vi "myRIO-1900 Customized FPGA.vi"() -> ()   [LabVIEW 2013]
doc: "This VI contains the NI myRIO FPGA shipping personality. This VI compiles and runs on the NI myRIO FPGA target. You can modify this VI to suit your application needs. National Instruments recommends that you only add new FPGA code to this VI and do not modify the existing code. This VI might not work correctly with the myRIO VIs if you modify the existing code."
uses:
  Sub VIs/Utilities/Start Boolean.ctl
  <vilib>/Platform/TimedLoop/XDataNode/timing_clust.ctl
  <vilib>/Platform/TimedLoop/XDataNode/nitl_modes.ctl
  <vilib>/Platform/TimedLoop/XDataNode/wakeup.ctl
  <vilib>/rvi/Emulation/niFpgaSctlEmulationGetInTimedLoop.vi
  <vilib>/rvi/Emulation/niFpgaEmulationReportErrorSimple.vi
  <vilib>/rvi/Emulation/niFpgaGetClockAttributes.vi
  <vilib>/rvi/Emulation/niFpgaCriticalErrorInLSC.vi
  <vilib>/rvi/eio/common/nirviEmuTemplateMethod_errors.vi
  <vilib>/rvi/eio/common/nirviEmuTemplatePropertyGet_noerrors.vi
  <vilib>/Platform/TimedLoop/XDataNode/XDataNode.xnode
  <vilib>/eio/EIONode/EIONode.xnode
  <vilib>/eio/EIOPropertyNode/EIOPropertyNode.xnode
  <vilib>/Platform/TimedLoop/XDataNode/XDNodeRunTimeDep.lvlib
  <vilib>/rvi/eio/common/nirviEmuTemplatePropertyGet_errors.vi
  <vilib>/rvi/eio/common/nirviEmuTemplatePropertySet_errors.vi
  <vilib>/rvi/eio/common/nirviEmuTemplatePropertySet_noerrors.vi
panel:
  out "Sonar Error 2":bool
  out "Sonar Timed Out 2":bool
  out "Sonar Reading 2":i32
  out "Sonar Error 1":bool
  out "Sonar Timed Out 1":bool
  out "Sonar Reading 1":i32
  out "Sonar Error 0":bool
  out "Sonar Timed Out 0":bool
  out "Sonar Reading 0":i32
  out "ACC.SCALE.WGHT":u16
  out "SYS.ACC_SCALE.RDY":bool
  out "AO.SYS.STAT":bool
  out "AI.B_1.WGHT":u32
  out "AO.B_0.WGHT":u32
  out "AO.B_1.WGHT":u32
  out "AO.B_0.OFST":u32
  out "AO.B_1.OFST":u32
  out "AO.A_0.WGHT":u32
  out "AO.A_1.WGHT":u32
  out "AO.C_0.WGHT":u32
  out "AO.C_1.WGHT":u32
  out "AO.AudioOut_L.WGHT":u32
  out "AO.AudioOut_R.WGHT":u32
  out "AO.A_0.OFST":u32
  out "AO.C_0.OFST":u32
  out "AO.C_1.OFST":u32
  out "AO.AudioOut_L.OFST":u32
  out "AO.AudioOut_R.OFST":u32
  out "AO.A_1.OFST":u32
  out "SYS.AO_SCALE.RDY":bool
  out "SYS.AI_SCALE.RDY":bool
  out "AI.A_1.OFST":u32
  out "AI.A_2.OFST":u32
  out "AI.A_3.OFST":u32
  out "AI.B_0.OFST":u32
  out "AI.B_1.OFST":u32
  out "AI.B_2.OFST":u32
  out "AI.B_3.OFST":u32
  out "AI.C_0.OFST":u32
  out "AI.C_1.OFST":u32
  out "AI.AudioIn_L.OFST":u32
  out "AI.AudioIn_R.OFST":u32
  out "AI.A_0.OFST":u32
  out "AI.AudioIn_R.WGHT":u32
  out "AI.AudioIn_L.WGHT":u32
  out "AI.C_1.WGHT":u32
  out "AI.C_0.WGHT":u32
  out "AI.B_3.WGHT":u32
  out "AI.B_2.WGHT":u32
  out "AI.B_0.WGHT":u32
  out "AI.A_3.WGHT":u32
  out "AI.A_2.WGHT":u32
  out "AI.A_1.WGHT":u32
  out "AI.A_0.WGHT":u32
  in  "DO.LED3:0":u8 format="%04b"
  out "ACC.Z.VAL":u16
  out "SYS.ACC.RDY":bool
  out "ACC.Y.VAL":u16
  out "ACC.X.VAL":u16
  in  "AO.SYS.GO":T1
  in  "AO.AudioOut_L.VAL":u16
  in  "AO.AudioOut_R.VAL":u16
  out "AI.AudioIn_L.VAL":u16
  out "AI.AudioIn_R.VAL":u16
  in  "DIO.B_15:8.OUT":u8 format="%08b"
  in  "DIO.B_15:8.DIR":u8 format="%08b"
  out "DIO.B_15:8.IN":u8 format="%08b"
  in  "DIO.A_15:8.DIR":u8 format="%08b"
  in  "DIO.A_15:8.OUT":u8 format="%08b"
  out "DIO.A_15:8.IN":u8 format="%08b"
  in  "PWM.C_0.MAX":u16
  in  "PWM.C_0.CMP":u16
  out "PWM.C_0.CNTR":u16
  in  "PWM.C_0.CNFG":u8 format="%08b"
  in  "PWM.C_0.CS":u8
  in  "PWM.C_1.MAX":u16
  in  "PWM.C_1.CMP":u16
  out "PWM.C_1.CNTR":u16
  in  "PWM.C_1.CNFG":u8 format="%08b"
  in  "PWM.C_1.CS":u8
  out "ENC.C_1.STAT":u8 format="%08b"
  out "ENC.C_1.CNTR":u32
  in  "ENC.C_1.CNFG":u8 format="%08b"
  out "ENC.C_0.STAT":u8 format="%08b"
  out "ENC.C_0.CNTR":u32
  in  "ENC.C_0.CNFG":u8 format="%08b"
  in  "SYS.SELECTA":u8 format="%08b"
  in  "SYS.SELECTC":u8 format="%08b"
  in  "SYS.SELECTB":u8 format="%08b"
  in  "AO.C_1.VAL":u16
  in  "AO.C_0.VAL":u16
  out "AI.C_0.VAL":u16
  out "AI.C_1.VAL":u16
  in  "DIO.C_7:0.OUT":u8 format="%08b"
  in  "DIO.C_7:0.DIR":u8 format="%08b"
  out "DIO.C_7:0.IN":u8 format="%08b"
  in  "DIO.A_7:0.DIR":u8 format="%08b"
  in  "DIO.A_7:0.OUT":u8 format="%08b"
  out "DIO.A_7:0.IN":u8 format="%08b"
  in  "PWM.B_0.CMP":u16
  in  "PWM.B_0.MAX":u16
  out "PWM.B_0.CNTR":u16
  in  "PWM.B_0.CNFG":u8 format="%08b"
  in  "PWM.B_0.CS":u8
  in  "PWM.B_1.CMP":u16
  in  "PWM.B_1.MAX":u16
  out "PWM.B_1.CNTR":u16
  in  "PWM.B_1.CNFG":u8 format="%08b"
  in  "PWM.B_1.CS":u8
  in  "PWM.B_2.CMP":u16
  in  "PWM.B_2.MAX":u16
  out "PWM.B_2.CNTR":u16
  in  "PWM.B_2.CNFG":u8 format="%08b"
  in  "PWM.B_2.CS":u8
  out "SYS.RDY":bool
  out "SYS.AI.RDY":bool
  in  "I2C.B.GO":T1
  in  "I2C.B.CNFG":u8 format="%08b"
  in  "I2C.B.DATO":u8
  out "I2C.B.DATI":u8
  in  "I2C.B.ADDR":u8 format="%08.0f"
  in  "I2C.B.CNTR":u8
  in  "I2C.B.CNTL":u8 format="%08b"
  out "I2C.B.STAT":u8 format="%08b"
  out "SPI.B.STAT":u8 format="%08b"
  in  "SPI.B.GO":T1
  out "SPI.A.STAT":u8 format="%08b"
  in  "SPI.A.GO":T1
  out "ENC.B.STAT":u8 format="%08b"
  out "ENC.A.STAT":u8 format="%08b"
  out "ENC.B.CNTR":u32
  out "ENC.A.CNTR":u32
  in  "ENC.B.CNFG":u8 format="%08b"
  in  "ENC.A.CNFG":u8 format="%08b"
  in  "SPI.B.DATO":u16
  out "SPI.B.DATI":u16
  in  "SPI.B.CNFG":u16 format="%016.0f"
  in  "SPI.B.CNT":u16
  in  "SPI.A.CNT":u16
  in  "SPI.A.CNFG":u16 format="%016b"
  out "SPI.A.DATI":u16
  in  "SPI.A.DATO":u16
  in  "PWM.A_0.MAX":u16
  in  "PWM.A_0.CMP":u16
  out "PWM.A_0.CNTR":u16
  in  "PWM.A_0.CNFG":u8 format="%08b"
  in  "PWM.A_0.CS":u8
  in  "PWM.A_1.CMP":u16
  in  "PWM.A_1.MAX":u16
  out "PWM.A_1.CNTR":u16
  in  "PWM.A_1.CNFG":u8 format="%08b"
  in  "PWM.A_1.CS":u8
  in  "PWM.A_2.CMP":u16
  in  "PWM.A_2.MAX":u16
  out "PWM.A_2.CNTR":u16
  in  "PWM.A_2.CNFG":u8 format="%08b"
  in  "PWM.A_2.CS":u8
  in  "DIO.B_7:0.OUT":u8 format="%08b"
  in  "DIO.B_7:0.DIR":u8 format="%08b"
  out "DIO.B_7:0.IN":u8 format="%08b"
  out "AI.A_0.VAL":u16
  out "AI.A_1.VAL":u16
  out "AI.A_2.VAL":u16
  out "AI.A_3.VAL":u16
  out "AI.B_0.VAL":u16
  out "AI.B_1.VAL":u16
  out "AI.B_2.VAL":u16
  out "AI.B_3.VAL":u16
  in  "AO.B_1.VAL":u16
  in  "AO.B_0.VAL":u16
  in  "AO.A_1.VAL":u16
  in  "AO.A_0.VAL":u16
  # "System"
  # "Onboard Devices"
  # "Connector A"
  # "Connector B"
  # "Connector C"
  # "Audio Connector"
  # "Accelerometer"
  # "Analog Input"
  # "Analog Output"
  # "Digital I/O"
  # "Counters / PWM"
  # "SPI Master"
  # "Analog Input"
  # "Analog Output"
  # "Digital I/O"
  # "Counters / PWM"
  # "SPI Master"
  # "Analog Input"
  # "Analog Output"
  # "Digital I/O"
  # "Counters / PWM"
  # "Analog Input"
  # "Encoders"
  # "Buttons & LEDs"
  # "I2C Master"
  # "I2C Master"
  # "Encoders"
  # "Encoders"
  # "Analog Output"
  # "IO Configuration"
  # "IO Configuration"
  # "IO Configuration"
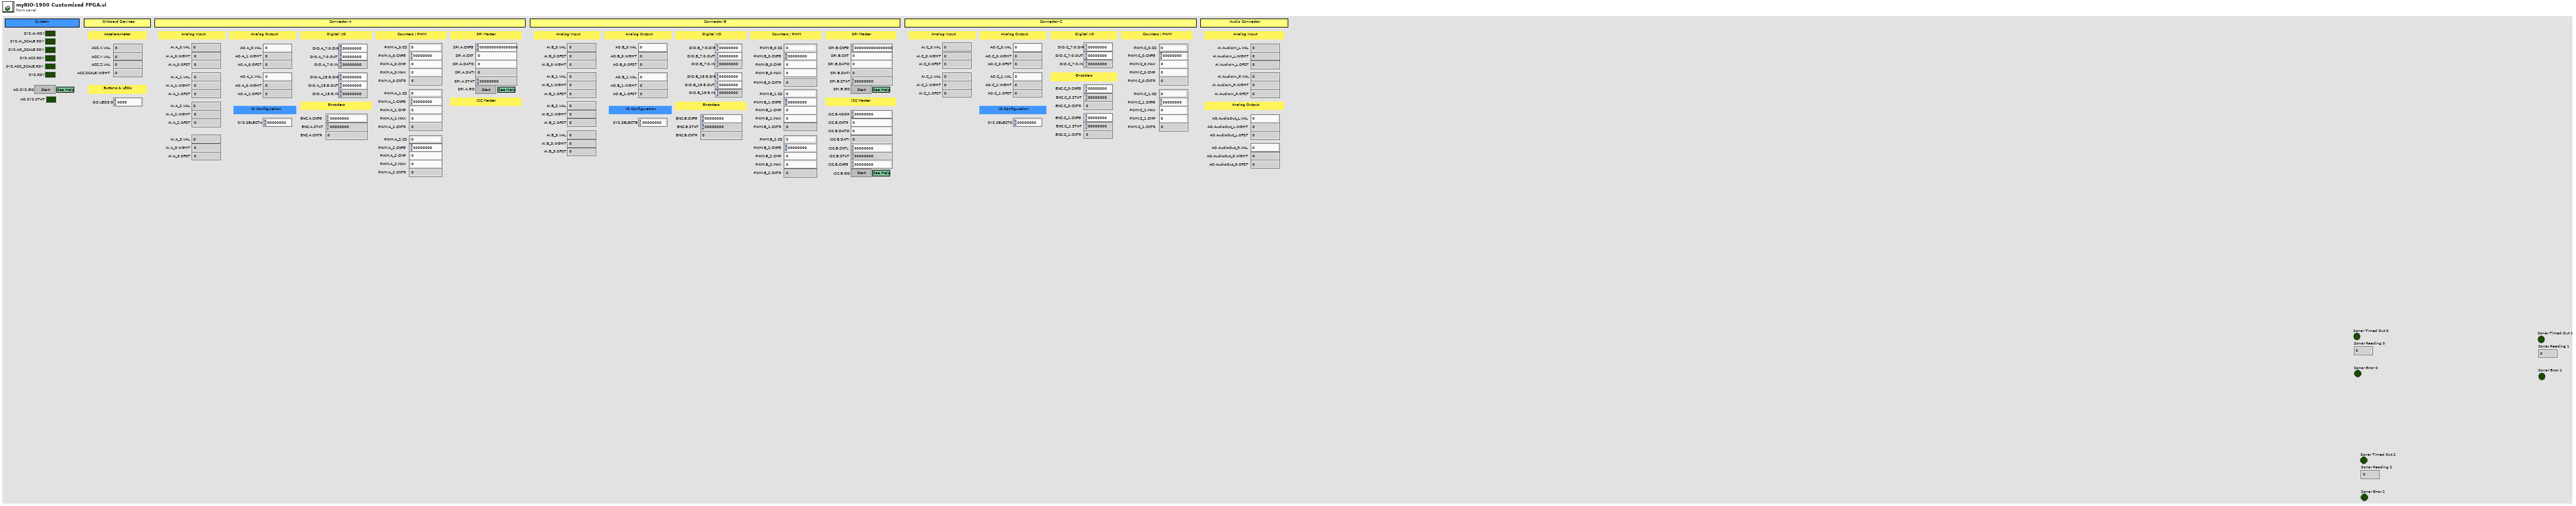
[diagram p1: front panel]
types:
  T1 = typedef "Start Boolean.ctl" = bool
  T2 = typedef "XDNodeRunTimeDep.lvlib/timing_clust.ctl" = cluster{"Expected End [f-1]":u64, "Actual End [f-1]":u64, "Finished Late? [f-1]":bool, "Expected End [i-1]":u64, "Actual End [i-1]":u64, "Finished Late? [i-1]":bool, "Expected Start [i]":u64, "Actual Start [i]":u64, "Expected Start [f]":u64, "Actual Start [f]":u64, "Source Name":string, "Structure Name":string, "Period":i64, "Deadline":i64, "Offset":i64, "Start":i64, "Priority":i32, "Timeout":i32, "Mode":T3, "Wakeup Reason":T4, "Error":errorcluster, "Source Type":string, "Secondary Source Type":string, "Global End Time":u64, "Global Start Time":u64, "Frame Duration":u64, "Iteration Duration":u64, "Assigned CPU":i32, "I/O Scan Engine Mode":u32}
  T3 = typedef "XDNodeRunTimeDep.lvlib/nitl_modes.ctl" = enum32{"No Change", "Process missed periods, maintain original phase", "Discard missed periods, maintain original phase", "Process missed periods, ignore original phase", "Discard missed periods, ignore original phase"}
  T4 = typedef "XDNodeRunTimeDep.lvlib/wakeup.ctl" = enum32{"Normal", "Aborted", "Asynchronous wakeup", "Timing source error", "Timed loop error", "Timeout"}
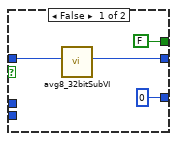
[diagram p2: hidden frame]
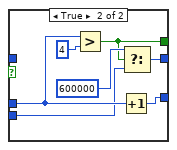
[diagram p3: hidden frame]
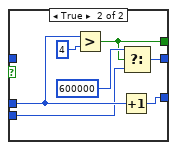
[diagram p4: hidden frame]
diagram:
  # "NOTE: The SYS.RDY boolean MUST exist and must become TRUE at some point otherwise the myRIO API will not function correctly."
  # "All DIO operations occur inside one single cycle timed loop (SCTL) since the IO is shared."
  # "The analog input scaling values are stored on the hardware. The RDY boolean should be checked before the values are used otherwise the analog input vlaues could be scaled incorrectly.\n\nAfter the first iteration of the while loop, all indicators have valid values."
  # "The analog output scaling values are stored on the hardware. The RDY boolean should be checked before the values are used otherwise the analog output vlaues could be scaled incorrectly.\n\nAfter the first iteration of the while loop, all indicators have valid values."
  # "The accelerometer nodes takes some time before the values can first be read (this is due to the time taken to read from the acceleromter). An iteration of the while loop will not complete until the accelerometer values have been read.\n\nAfter the first iteration of the while loop, all indicators have valid values."
  # "The onboard accelerometer has a range of +/- 8g which translates to 256 bits/g. The scaling weight is hardcoded in the FPGA to allow for future updates with minimal changes in the myRIO code. The RDY boolean should be checked before the values are used otherwise the analog output vlaues could be scaled incorrectly.\n\nAfter the first iteration of the while loop, all indicators have valid values."
  # "Onboard Accelerometer Scaling"
  # "Analog Output Scaling Constants"
  # "Analog Input Scaling Constants"
  # "Onboard Accelerometer"
  # "Onboard DIO"
  # "Connector B DIO"
  # "There is some delay between when the FPGA code starts and the analog inputs, accelerometer, and scaling values outputs are valid. If the host wants to ensure that there are valid values in theses registers it should wait for each subsystem to finish its initialization process. \n\nWhen all subsystems have finished initializinig, the SYS.RDY indicator will be true, which can be polled by the host to determine the status of the FPGA. Alternatively, the host can poll the individual SYS.xx.RDY indicators to determine the status of the individual subsystems.\n\nThis loop continues indefinitely, essentially making SYS.RDY a read-only register."
  # "The analog input nodes takes some time before the values can first be read (this is due to the time taken to setup the ADC and convert the first reading). An iteration of the while loop will not complete until all the analog input channels have been sampled.\n\nAfter the first iteration of the while loop, all indicators have valid values."
  # "Note: On some hardware a \"ghosting effect\" may occur on any unconnected AI channels. For example, if channel AI0 is connected and channels AI1 - AI7 are not connected the the value read at AI0 may be seen on indicators AI1 - AI7. This is common for hardware that use a multiplexed (MUXed) Analog-to-Digital converter (ADC) since the input analog signal is used to charge a capacitor which does not discharge before the unconnected channel is read.\n\n\"Ghosting\" effect can be hidden be using an mask register which will be used to decide when the indicator should be updated."
  # "The analog output nodes take some time before values are written to the pins. The GO and STAT registers are used to handshake between the FPGA and host. When the host wants the values to be written it sets the GO register to true. If the host reads the STAT register before setting GO, it can then wait for the STAT register value to invert which will tell the host that the output values have been written."
  # "Connector A DIO"
  # "Connector C  DIO"
  # "Host Synchronization"
  # "Analog Output"
  # "Analog Input"
  n1 = while {
    stop <- FALSE stop-if-true
    n2 = local read "SYS.ACC_SCALE.RDY"() -> (w10:bool)
    n3 = local read "SYS.AO_SCALE.RDY"() -> (w11:bool)
    n4 = local read "SYS.AI_SCALE.RDY"() -> (w12:bool)
    n5 = local read "SYS.ACC.RDY"() -> (w13:bool)
    n6 = local read "SYS.AI.RDY"() -> (w15:bool)
    n7 = Compound Arithmetic op=AND(w15, w13, w12, w11, w10) -> (→"SYS.RDY":bool)
  }
  n8 = while {
    i -> [w27]
    stop <- FALSE stop-if-true
    n9 = xnode "FPGA I/O Node"() -> ("ConnectorA/AI0"=→"AI.A_0.VAL":u16, "ConnectorA/AI1"=→"AI.A_1.VAL":u16, "ConnectorA/AI2"=→"AI.A_2.VAL":u16, "ConnectorA/AI3"=→"AI.A_3.VAL":u16, "ConnectorB/AI0"=→"AI.B_0.VAL":u16, "ConnectorB/AI1"=→"AI.B_1.VAL":u16, "ConnectorB/AI2"=→"AI.B_2.VAL":u16, "ConnectorB/AI3"=→"AI.B_3.VAL":u16, "ConnectorC/AI0"=w21:i16, "ConnectorC/AI1"=w20:i16, "AudioIn/Left"=w19:i16, "AudioIn/Right"=w18:i16)  [unwired: 12 in, 12 out]
    n10 = Greater Than 0?(x=w27) -> (x > 0?=→"SYS.AI.RDY":bool)
    n11 = To Unsigned Word Integer(number=w21) -> (unsigned 16bit integer=→"AI.C_0.VAL":u16)
    n12 = To Unsigned Word Integer(number=w20) -> (unsigned 16bit integer=→"AI.C_1.VAL":u16)
    n13 = To Unsigned Word Integer(number=w19) -> (unsigned 16bit integer=→"AI.AudioIn_L.VAL":u16)
    n14 = To Unsigned Word Integer(number=w18) -> (unsigned 16bit integer=→"AI.AudioIn_R.VAL":u16)
  }
  n15 = while {
    i -> [w37]
    stop <- FALSE stop-if-true
    n16 = Greater Than 0?(x=w37) -> (x > 0?=→"SYS.AI_SCALE.RDY":bool)
    n17 = xnode "FPGA I/O Property Node"("FPGA I/O In"=refnum<k21> "ConnectorA/AI0" ("FPGA I/O")) -> ("LSB Weight"=→"AI.A_0.WGHT":u32, "Offset"=w62:i32)  [unwired: 1 out]
    n18 = xnode "FPGA I/O Property Node"("FPGA I/O In"=refnum<k21> "ConnectorA/AI1" ("FPGA I/O")) -> ("LSB Weight"=→"AI.A_1.WGHT":u32, "Offset"=w50:i32)  [unwired: 1 out]
    n19 = xnode "FPGA I/O Property Node"("FPGA I/O In"=refnum<k21> "ConnectorA/AI2" ("FPGA I/O")) -> ("LSB Weight"=→"AI.A_2.WGHT":u32, "Offset"=w59:i32)  [unwired: 1 out]
    n20 = xnode "FPGA I/O Property Node"("FPGA I/O In"=refnum<k21> "ConnectorA/AI3" ("FPGA I/O")) -> ("LSB Weight"=→"AI.A_3.WGHT":u32, "Offset"=w58:i32)  [unwired: 1 out]
    n21 = xnode "FPGA I/O Property Node"("FPGA I/O In"=refnum<k21> "ConnectorB/AI0" ("FPGA I/O")) -> ("LSB Weight"=→"AI.B_0.WGHT":u32, "Offset"=w57:i32)  [unwired: 1 out]
    n22 = xnode "FPGA I/O Property Node"("FPGA I/O In"=refnum<k21> "ConnectorB/AI1" ("FPGA I/O")) -> ("LSB Weight"=→"AI.B_1.WGHT":u32, "Offset"=w56:i32)  [unwired: 1 out]
    n23 = xnode "FPGA I/O Property Node"("FPGA I/O In"=refnum<k21> "ConnectorB/AI2" ("FPGA I/O")) -> ("LSB Weight"=→"AI.B_2.WGHT":u32, "Offset"=w55:i32)  [unwired: 1 out]
    n24 = xnode "FPGA I/O Property Node"("FPGA I/O In"=refnum<k21> "ConnectorB/AI3" ("FPGA I/O")) -> ("LSB Weight"=→"AI.B_3.WGHT":u32, "Offset"=w54:i32)  [unwired: 1 out]
    n25 = xnode "FPGA I/O Property Node"("FPGA I/O In"=refnum<k21> "ConnectorC/AI0" ("FPGA I/O")) -> ("LSB Weight"=→"AI.C_0.WGHT":u32, "Offset"=w53:i32)  [unwired: 1 out]
    n26 = xnode "FPGA I/O Property Node"("FPGA I/O In"=refnum<k21> "ConnectorC/AI1" ("FPGA I/O")) -> ("LSB Weight"=→"AI.C_1.WGHT":u32, "Offset"=w52:i32)  [unwired: 1 out]
    n27 = xnode "FPGA I/O Property Node"("FPGA I/O In"=refnum<k21> "AudioIn/Left" ("FPGA I/O")) -> ("LSB Weight"=→"AI.AudioIn_L.WGHT":u32, "Offset"=w51:i32)  [unwired: 1 out]
    n28 = xnode "FPGA I/O Property Node"("FPGA I/O In"=refnum<k21> "AudioIn/Right" ("FPGA I/O")) -> ("LSB Weight"=→"AI.AudioIn_R.WGHT":u32, "Offset"=w61:i32)  [unwired: 1 out]
    n29 = To Unsigned Long Integer(number=w62) -> (unsigned 32bit integer=→"AI.A_0.OFST":u32)
    n30 = To Unsigned Long Integer(number=w50) -> (unsigned 32bit integer=→"AI.A_1.OFST":u32)
    n31 = To Unsigned Long Integer(number=w59) -> (unsigned 32bit integer=→"AI.A_2.OFST":u32)
    n32 = To Unsigned Long Integer(number=w58) -> (unsigned 32bit integer=→"AI.A_3.OFST":u32)
    n33 = To Unsigned Long Integer(number=w57) -> (unsigned 32bit integer=→"AI.B_0.OFST":u32)
    n34 = To Unsigned Long Integer(number=w56) -> (unsigned 32bit integer=→"AI.B_1.OFST":u32)
    n35 = To Unsigned Long Integer(number=w55) -> (unsigned 32bit integer=→"AI.B_2.OFST":u32)
    n36 = To Unsigned Long Integer(number=w54) -> (unsigned 32bit integer=→"AI.B_3.OFST":u32)
    n37 = To Unsigned Long Integer(number=w53) -> (unsigned 32bit integer=→"AI.C_0.OFST":u32)
    n38 = To Unsigned Long Integer(number=w52) -> (unsigned 32bit integer=→"AI.C_1.OFST":u32)
    n39 = To Unsigned Long Integer(number=w51) -> (unsigned 32bit integer=→"AI.AudioIn_L.OFST":u32)
    n40 = To Unsigned Long Integer(number=w61) -> (unsigned 32bit integer=→"AI.AudioIn_R.OFST":u32)
  }
  n41 = while {
    stop <- FALSE stop-if-true
    n42 = feedback #1(FALSE) -> (w88:bool)
    n43 = case shown="True" "AO.SYS.GO" {
      tunnel: "AO.C_0.VAL" -> [_ w110]
      tunnel: "AO.C_1.VAL" -> [_ w109]
      tunnel: "AO.A_0.VAL" -> [_ w114]
      tunnel: "AO.A_1.VAL" -> [_ w113]
      tunnel: "AO.B_0.VAL" -> [_ w112]
      tunnel: "AO.B_1.VAL" -> [_ w111]
      tunnel: "AO.AudioOut_L.VAL" -> [_ w106]
      tunnel: "AO.AudioOut_R.VAL" -> [_ w105]
      tunnel: w88 -> [w99 w102]
      tunnel: [w99 w100] -> w86
      frame False {
      }
      frame True {
        n44 = To Word Integer(number=w110) -> (16bit integer=w108:i16)
        n45 = To Word Integer(number=w109) -> (16bit integer=w107:i16)
        n46 = To Word Integer(number=w106) -> (16bit integer=w104:i16)
        n47 = To Word Integer(number=w105) -> (16bit integer=w103:i16)
        n48 = flat-sequence {
          tunnel: w114 -> [w123]
          tunnel: w113 -> [w122]
          tunnel: w112 -> [w121]
          tunnel: w111 -> [w120]
          tunnel: w108 -> [w119]
          tunnel: w107 -> [w118]
          tunnel: w104 -> [w117]
          tunnel: w103 -> [w116]
          tunnel: w102 -> [w115]
          tunnel: [w115] -> w101
          tunnel: w101 -> [w125]
          tunnel: [w124] -> w100
          frame #0 {
            n49 = xnode "FPGA I/O Node"("ConnectorA/AO0"=w123, "ConnectorA/AO1"=w122, "ConnectorB/AO0"=w121, "ConnectorB/AO1"=w120, "ConnectorC/AO0"=w119, "ConnectorC/AO1"=w118, "AudioOut/Left"=w117, "AudioOut/Right"=w116) -> ()  [unwired: 8 in, 8 out]
          }
          frame #1 {
            n50 = Not(x=w125) -> (.not. x?=w124:bool)
          }
        }
      }
    }
    "AO.SYS.STAT" <- w86
    n51 = feedback-in #1(w86) -> ()
  }
  n52 = while {
    i -> [w147]
    stop <- FALSE stop-if-true
    n53 = Greater Than 0?(x=w147) -> (x > 0?=→"SYS.AO_SCALE.RDY":bool)
    n54 = xnode "FPGA I/O Property Node"("FPGA I/O In"=refnum<k21> "ConnectorA/AO0" ("FPGA I/O")) -> ("LSB Weight"=→"AO.A_0.WGHT":u32, "Offset"=w158:i32)  [unwired: 1 out]
    n55 = xnode "FPGA I/O Property Node"("FPGA I/O In"=refnum<k21> "ConnectorA/AO1" ("FPGA I/O")) -> ("LSB Weight"=→"AO.A_1.WGHT":u32, "Offset"=w150:i32)  [unwired: 1 out]
    n56 = xnode "FPGA I/O Property Node"("FPGA I/O In"=refnum<k21> "ConnectorB/AO0" ("FPGA I/O")) -> ("LSB Weight"=→"AO.B_0.WGHT":u32, "Offset"=w156:i32)  [unwired: 1 out]
    n57 = xnode "FPGA I/O Property Node"("FPGA I/O In"=refnum<k21> "ConnectorB/AO1" ("FPGA I/O")) -> ("LSB Weight"=→"AO.B_1.WGHT":u32, "Offset"=w155:i32)  [unwired: 1 out]
    n58 = xnode "FPGA I/O Property Node"("FPGA I/O In"=refnum<k21> "ConnectorC/AO0" ("FPGA I/O")) -> ("LSB Weight"=→"AO.C_0.WGHT":u32, "Offset"=w154:i32)  [unwired: 1 out]
    n59 = xnode "FPGA I/O Property Node"("FPGA I/O In"=refnum<k21> "ConnectorC/AO1" ("FPGA I/O")) -> ("LSB Weight"=→"AO.C_1.WGHT":u32, "Offset"=w153:i32)  [unwired: 1 out]
    n60 = xnode "FPGA I/O Property Node"("FPGA I/O In"=refnum<k21> "AudioOut/Left" ("FPGA I/O")) -> ("LSB Weight"=→"AO.AudioOut_L.WGHT":u32, "Offset"=w152:i32)  [unwired: 1 out]
    n61 = xnode "FPGA I/O Property Node"("FPGA I/O In"=refnum<k21> "AudioOut/Right" ("FPGA I/O")) -> ("LSB Weight"=→"AO.AudioOut_R.WGHT":u32, "Offset"=w151:i32)  [unwired: 1 out]
    n62 = To Unsigned Long Integer(number=w158) -> (unsigned 32bit integer=→"AO.A_0.OFST":u32)
    n63 = To Unsigned Long Integer(number=w150) -> (unsigned 32bit integer=→"AO.A_1.OFST":u32)
    n64 = To Unsigned Long Integer(number=w156) -> (unsigned 32bit integer=→"AO.B_0.OFST":u32)
    n65 = To Unsigned Long Integer(number=w155) -> (unsigned 32bit integer=→"AO.B_1.OFST":u32)
    n66 = To Unsigned Long Integer(number=w154) -> (unsigned 32bit integer=→"AO.C_0.OFST":u32)
    n67 = To Unsigned Long Integer(number=w153) -> (unsigned 32bit integer=→"AO.C_1.OFST":u32)
    n68 = To Unsigned Long Integer(number=w152) -> (unsigned 32bit integer=→"AO.AudioOut_L.OFST":u32)
    n69 = To Unsigned Long Integer(number=w151) -> (unsigned 32bit integer=→"AO.AudioOut_R.OFST":u32)
  }
  n70 = while {
    i -> [w165]
    stop <- FALSE stop-if-true
    # "E-stop"
    # "The onboard accelerometer has a range of +/-8g which translates to 256 bits / g. The scaling weight is hardcoded in the FPGA to"
    n71 = xnode "FPGA I/O Node"() -> ("Button0"=w162:bool)  [unwired: 1 in, 1 out]
    n72 = Greater Than 0?(x=w165) -> (x > 0?=→"SYS.ACC_SCALE.RDY":bool)
    n73 = call "RisingEdgeSubVI.vi"("Signal In"=w162) -> ("Rising Edge"=w161:bool)  [unwired: 10 in]
    n74 = case shown="True" w161 {
      frame False {
      }
      frame True {
        n75 = call <vilib>:"niFPGA Interrupt.vi"("Wait Until Cleared (F)"=FALSE ("Wait Until Cleared"), "IRQ Number (0)"=u8 0 ("IRQ Number")) -> ()  [unwired: 1 in]
      }
    }
    "ACC.SCALE.WGHT" <- u16 256 ("ACC.SCALE.WGHT")
  }
  n76 = node-c288() -> (w2:T2)  [unwired: 1 in]
  n77 = timed-loop {
    timing: w2 -> [_]
    timing-out: [_] -> w1
    stop <- _ stop-if-true
    n78 = Number To Boolean Array(number="DO.LED3:0") -> (Boolean array=w173:bool[])
    n79 = Index Array(array=w173) -> (element #1=w172:bool, element #2=w171:bool, element #3=w170:bool, element #4=w169:bool)  [unwired: 4 in]
    n80 = xnode "FPGA I/O Node"("LED0"=w172, "LED1"=w171, "LED2"=w170, "LED3"=w169) -> ()  [unwired: 4 in, 4 out]
  }
  n81 = while {
    i -> [w181]
    stop <- FALSE stop-if-true
    n82 = xnode "FPGA I/O Node"() -> ("AccelerationX"=w184:i16, "AccelerationY"=w183:i16, "AccelerationZ"=w182:i16)  [unwired: 3 in, 3 out]
    n83 = Greater Than 0?(x=w181) -> (x > 0?=→"SYS.ACC.RDY":bool)
    n84 = To Unsigned Word Integer(number=w184) -> (unsigned 16bit integer=→"ACC.X.VAL":u16)
    n85 = To Unsigned Word Integer(number=w183) -> (unsigned 16bit integer=→"ACC.Y.VAL":u16)
    n86 = To Unsigned Word Integer(number=w182) -> (unsigned 16bit integer=→"ACC.Z.VAL":u16)
  }
  n87 = node-c288(w1) -> ()
  n88 = node-c288() -> (w6:T2)  [unwired: 1 in]
  n89 = timed-loop {
    timing: w6 -> [_]
    timing-out: [_] -> w5
    stop <- FALSE stop-if-true
    w197 = FALSE ("element")
    # "DIO / Encoder"
    # "DIO / I2C Master"
    # "DIO / PWM"
    # "DIO"
    # "DIO"
    # "DIO/ SPI Master"
    n90 = call "Split HDC Bank1 DIO.vi"("IN 7:0"="DIO.A_7:0.OUT") -> ("OUT 3:0"=w191:fxp<+,4,4>, "OUT 4"=w195:bool, "OUT 7:5"=w260:fxp<+,3,3>)
    n91 = call "Split HDC Bank1 DIO.vi"("IN 7:0"="DIO.A_7:0.DIR") -> ("OUT 3:0"=w192:fxp<+,4,4>, "OUT 4"=w194:bool, "OUT 7:5"=w259:fxp<+,3,3>)
    n92 = call "Split HDC Function Select.vi"("IN 7:0"="SYS.SELECTA") -> ("OUT 1:0"=w219:fxp<+,2,2>, "OUT 2"=w218:bool, "OUT 3"=w217:bool, "OUT 4"=w216:bool, "OUT 5"=w215:bool)  [unwired: 1 out]
    n93 = call "DIO_SPI.vi"("DIO.2:0.OUT"=w260, "DIO.2:0.DIR"=w259, "SPI.CNT"="SPI.A.CNT", "SPI.CNFG"="SPI.A.CNFG", "SPI.DATO"="SPI.A.DATO", "SPI.GO"="SPI.A.GO", "DIO.2/SPI.MOSI Refnum"=refnum<k21> "ConnectorA/DIO7" ("DIO.2/SPI.SCLK"), "SELECT.1:0"=w219, "DIO.1/SPI.MISO Refnum"=refnum<k21> "ConnectorA/DIO6" ("DIO.1/SPI.MOSI"), "DIO.0/SPI.SCLK Refnum"=refnum<k21> "ConnectorA/DIO5" ("DIO.0/SPI.MISO")) -> ("DIO.2:0.IN"=w242:fxp<+,3,3>, "SPI.DATI"=→"SPI.A.DATI":u16, "SPI.STAT"=→"SPI.A.STAT":u8)  [unwired: 7 in]
    n94 = call "DIO 1-bit.vi"("DIR"=w194, "OUT"=w195, "DIO Refnum"=refnum<k21> "ConnectorA/DIO4") -> ("IN"=w193:bool)  [unwired: 8 in]
    n95 = call "3DIO.vi"("DIO3 Refnum"=refnum<k21> "ConnectorA/DIO3", "DIO1 Refnum"=refnum<k21> "ConnectorA/DIO1", "DIR 3:0"=w192, "OUT 3:0"=w191, "DIO0 Refnum"=refnum<k21> "ConnectorA/DIO0") -> ("IN 3:0"=w187:fxp<+,4,4>)  [unwired: 6 in]
    n96 = call "Join HDC Bank1 DIO.vi"("IN 7:5"=w242, "IN 4"=w193, "IN 3:0"=w187) -> ("OUT 7:0"=→"DIO.A_7:0.IN":u8)
    n97 = call "Split HDC Bank2 DIO.vi"("IN 7:0"="DIO.A_15:8.DIR") -> ("OUT 4:3"=w207:fxp<+,2,2>, "OUT 2"=w209:bool, "OUT 0"=w212:bool, "OUT 1"=w211:bool)  [unwired: 2 in, 2 out]
    n98 = call "Split HDC Bank2 DIO.vi"("IN 7:0"="DIO.A_15:8.OUT") -> ("OUT 4:3"=w208:fxp<+,2,2>, "OUT 2"=w210:bool, "OUT 0"=w214:bool, "OUT 1"=w213:bool)  [unwired: 2 in, 2 out]
    n99 = call "DIO_PWM.vi"("DIO.OUT"=w214, "DIO.DIR"=w212, "PWM.CS"="PWM.A_0.CS", "PWM.CNFG"="PWM.A_0.CNFG", "PWM.CMP"="PWM.A_0.CMP", "PWM.MAX"="PWM.A_0.MAX", "DIO/PWM"=refnum<k21> "ConnectorA/DIO8", "SELECT"=w218) -> ("DIO.IN"=w201:bool, "PWM.CNTR"=→"PWM.A_0.CNTR":u16)  [unwired: 10 in]
    n100 = call "DIO_PWM.vi"("DIO.OUT"=w213, "DIO.DIR"=w211, "PWM.CS"="PWM.A_1.CS", "PWM.CNFG"="PWM.A_1.CNFG", "PWM.CMP"="PWM.A_1.CMP", "PWM.MAX"="PWM.A_1.MAX", "DIO/PWM"=refnum<k21> "ConnectorA/DIO9", "SELECT"=w217) -> ("DIO.IN"=w200:bool, "PWM.CNTR"=→"PWM.A_1.CNTR":u16)  [unwired: 10 in]
    n101 = call "DIO_PWM.vi"("DIO.OUT"=w210, "DIO.DIR"=w209, "PWM.CS"="PWM.A_2.CS", "PWM.CNFG"="PWM.A_2.CNFG", "PWM.CMP"="PWM.A_2.CMP", "PWM.MAX"="PWM.A_2.MAX", "DIO/PWM"=refnum<k21> "ConnectorA/DIO10", "SELECT"=w216) -> ("DIO.IN"=w199:bool, "PWM.CNTR"=→"PWM.A_2.CNTR":u16)  [unwired: 10 in]
    n102 = call "DIO_Encoder.vi"("DIO.1:0.OUT"=w208, "DIO.1:0.DIR"=w207, "QE.CNFG"="ENC.A.CNFG", "DIO.1/QE.B"=refnum<k21> "ConnectorA/DIO12", "SELECT"=w215, "DIO.0/QE.A"=refnum<k21> "ConnectorA/DIO11") -> ("DIO.1:0.IN"=w198:fxp<+,2,2>, "QE.CNTR"=→"ENC.A.CNTR":u32, "QE.STAT"=→"ENC.A.STAT":u8)  [unwired: 11 in]
    n103 = Number To Boolean Array(number=w198) -> (Boolean array=w205:bool[])
    n104 = Index Array(array=w205) -> (element #1=w204:bool, element #2=w203:bool)  [unwired: 2 in]
    n105 = Build Array(w201, w200, w199, w204, w203, w197, w197, w197) -> (w206:bool[])
    n106 = Boolean Array To Number(Boolean array=w206) -> (number=→"DIO.A_15:8.IN":u8)
  }
  n107 = while {
    stop <- FALSE stop-if-true
    n108 = call "SonarK.vi"("FPGA I/O In"=refnum<k21> "ConnectorA/DIO13") -> ("Error in System"=→"Sonar Error 0":bool, "Timed Out"=w267:bool, "Output"=w266:i32)  [unwired: 8 in]
    n109 = feedback #2() -> (w265:i32)  [unwired: 1 in]
    n110 = feedback #3() -> (w263:u16)  [unwired: 1 in]
    n111 = case shown="False" w267 {
      tunnel: w266 -> [w275 _]
      tunnel: [w274 w279] -> w268
      tunnel: w265 -> [_ w280]
      tunnel: [u16 0 w283] -> w264
      tunnel: w263 -> [_ w282]
      tunnel: [FALSE w277] -> w270
      frame False {
        n112 = call "avg8_32bitSubVI.vi"("Input"=w275) -> ("Output"=w274:i32)  [unwired: 10 in]
      }
      frame True {
        n113 = Greater?(x=w282, y=u16 4) -> (0:w277:bool)
        n114 = Increment(x=w282) -> (x+1=w283:u16)
        n115 = Select(t=600000, s=w277, f=w280) -> (s? t:f=w279:i32)
      }
    }
    "Sonar Timed Out 0" <- w270
    "Sonar Reading 0" <- w268
    n116 = feedback-in #2(w268) -> ()
    n117 = feedback-in #3(w264) -> ()
  }
  n118 = while {
    stop <- FALSE stop-if-true
    n119 = call "SonarK.vi"("FPGA I/O In"=refnum<k21> "ConnectorA/DIO15") -> ("Error in System"=→"Sonar Error 2":bool, "Timed Out"=w288:bool, "Output"=w287:i32)  [unwired: 8 in]
    n120 = feedback #4() -> (w284:u16)  [unwired: 1 in]
    n121 = feedback #5() -> (w286:i32)  [unwired: 1 in]
    n122 = case shown="True" w288 {
      tunnel: w287 -> [w296 _]
      tunnel: [w295 w300] -> w290
      tunnel: w286 -> [_ w301]
      tunnel: [u16 0 w304] -> w285
      tunnel: w284 -> [_ w303]
      tunnel: [FALSE w298] -> w291
      frame False {
        n123 = call "avg8_32bitSubVI.vi"("Input"=w296) -> ("Output"=w295:i32)  [unwired: 10 in]
      }
      frame True {
        n124 = Greater?(x=w303, y=u16 4) -> (0:w298:bool)
        n125 = Increment(x=w303) -> (x+1=w304:u16)
        n126 = Select(t=600000, s=w298, f=w301) -> (s? t:f=w300:i32)
      }
    }
    "Sonar Timed Out 2" <- w291
    "Sonar Reading 2" <- w290
    n127 = feedback-in #4(w285) -> ()
    n128 = feedback-in #5(w290) -> ()
  }
  n129 = while {
    stop <- FALSE stop-if-true
    n130 = call "SonarK.vi"("FPGA I/O In"=refnum<k21> "ConnectorA/DIO14") -> ("Error in System"=→"Sonar Error 1":bool, "Timed Out"=w309:bool, "Output"=w308:i32)  [unwired: 8 in]
    n131 = feedback #6() -> (w305:u16)  [unwired: 1 in]
    n132 = feedback #7() -> (w307:i32)  [unwired: 1 in]
    n133 = case shown="False" w309 {
      tunnel: w308 -> [w317 _]
      tunnel: [w316 w321] -> w310
      tunnel: w307 -> [_ w322]
      tunnel: [u16 0 w325] -> w306
      tunnel: w305 -> [_ w324]
      tunnel: [FALSE w319] -> w312
      frame False {
        n134 = call "avg8_32bitSubVI.vi"("Input"=w317) -> ("Output"=w316:i32)  [unwired: 10 in]
      }
      frame True {
        n135 = Greater?(x=w324, y=u16 4) -> (0:w319:bool)
        n136 = Increment(x=w324) -> (x+1=w325:u16)
        n137 = Select(t=600000, s=w319, f=w322) -> (s? t:f=w321:i32)
      }
    }
    "Sonar Timed Out 1" <- w312
    "Sonar Reading 1" <- w310
    n138 = feedback-in #6(w306) -> ()
    n139 = feedback-in #7(w310) -> ()
  }
  n140 = node-c288(w5) -> ()
  n141 = node-c288() -> (w4:T2)  [unwired: 1 in]
  n142 = timed-loop {
    timing: w4 -> [_]
    timing-out: [_] -> w3
    stop <- FALSE stop-if-true
    # "DIO / Encoder"
    # "DIO / I2C Master"
    # "DIO / PWM"
    # "DIO"
    # "DIO"
    # "DIO/ SPI Master"
    n143 = call "Split HDC Bank1 DIO.vi"("IN 7:0"="DIO.B_7:0.OUT") -> ("OUT 3:0"=w414:fxp<+,4,4>, "OUT 4"=w412:bool, "OUT 7:5"=w410:fxp<+,3,3>)
    n144 = call "Split HDC Bank1 DIO.vi"("IN 7:0"="DIO.B_7:0.DIR") -> ("OUT 3:0"=w413:fxp<+,4,4>, "OUT 4"=w411:bool, "OUT 7:5"=w409:fxp<+,3,3>)
    n145 = call "Split HDC Function Select.vi"("IN 7:0"="SYS.SELECTB") -> ("OUT 1:0"=w386:fxp<+,2,2>, "OUT 7"=w381:bool, "OUT 2"=w385:bool, "OUT 3"=w384:bool, "OUT 4"=w383:bool, "OUT 5"=w382:bool)
    n146 = call "DIO 4-bit.vi"("DIO0 Refnum"=refnum<k21> "ConnectorB/DIO0", "DIO1 Refnum"=refnum<k21> "ConnectorB/DIO1", "DIO2 Refnum"=refnum<k21> "ConnectorB/DIO2", "DIR 3:0"=w413, "OUT 3:0"=w414, "DIO3 Refnum"=refnum<k21> "ConnectorB/DIO3") -> ("IN 3:0"=w392:fxp<+,4,4>)  [unwired: 5 in]
    n147 = call "DIO 1-bit.vi"("DIR"=w411, "OUT"=w412, "DIO Refnum"=refnum<k21> "ConnectorB/DIO4") -> ("IN"=w391:bool)  [unwired: 8 in]
    n148 = call "DIO_SPI.vi"("DIO.2:0.OUT"=w410, "DIO.2:0.DIR"=w409, "SPI.CNT"="SPI.B.CNT", "SPI.CNFG"="SPI.B.CNFG", "SPI.DATO"="SPI.B.DATO", "SPI.GO"="SPI.B.GO", "DIO.2/SPI.MOSI Refnum"=refnum<k21> "ConnectorB/DIO7" ("DIO.2/SPI.SCLK"), "SELECT.1:0"=w386, "DIO.1/SPI.MISO Refnum"=refnum<k21> "ConnectorB/DIO6" ("DIO.1/SPI.MOSI"), "DIO.0/SPI.SCLK Refnum"=refnum<k21> "ConnectorB/DIO5" ("DIO.0/SPI.MISO")) -> ("DIO.2:0.IN"=w390:fxp<+,3,3>, "SPI.DATI"=→"SPI.B.DATI":u16, "SPI.STAT"=→"SPI.B.STAT":u8)  [unwired: 7 in]
    n149 = call "Join HDC Bank1 DIO.vi"("IN 7:5"=w390, "IN 4"=w391, "IN 3:0"=w392) -> ("OUT 7:0"=→"DIO.B_7:0.IN":u8)
    n150 = call "Split HDC Bank2 DIO.vi"("IN 7:0"="DIO.B_15:8.OUT") -> ("OUT 5"=w337:bool, "OUT 7:6"=w389:fxp<+,2,2>, "OUT 4:3"=w338:fxp<+,2,2>, "OUT 2"=w339:bool, "OUT 0"=w341:bool, "OUT 1"=w340:bool)  [unwired: 2 in]
    n151 = call "Split HDC Bank2 DIO.vi"("IN 7:0"="DIO.B_15:8.DIR") -> ("OUT 5"=w332:bool, "OUT 7:6"=w388:fxp<+,2,2>, "OUT 4:3"=w333:fxp<+,2,2>, "OUT 2"=w334:bool, "OUT 0"=w336:bool, "OUT 1"=w335:bool)  [unwired: 2 in]
    n152 = call "DIO_PWM.vi"("DIO.OUT"=w341, "DIO.DIR"=w336, "PWM.CS"="PWM.B_0.CS", "PWM.CNFG"="PWM.B_0.CNFG", "PWM.CMP"="PWM.B_0.CMP", "PWM.MAX"="PWM.B_0.MAX", "DIO/PWM"=refnum<k21> "ConnectorB/DIO8", "SELECT"=w385) -> ("DIO.IN"=w331:bool, "PWM.CNTR"=→"PWM.B_0.CNTR":u16)  [unwired: 10 in]
    n153 = call "DIO_PWM.vi"("DIO.OUT"=w340, "DIO.DIR"=w335, "PWM.CS"="PWM.B_1.CS", "PWM.CNFG"="PWM.B_1.CNFG", "PWM.CMP"="PWM.B_1.CMP", "PWM.MAX"="PWM.B_1.MAX", "DIO/PWM"=refnum<k21> "ConnectorB/DIO9", "SELECT"=w384) -> ("DIO.IN"=w330:bool, "PWM.CNTR"=→"PWM.B_1.CNTR":u16)  [unwired: 10 in]
    n154 = call "DIO_PWM.vi"("DIO.OUT"=w339, "DIO.DIR"=w334, "PWM.CS"="PWM.B_2.CS", "PWM.CNFG"="PWM.B_2.CNFG", "PWM.CMP"="PWM.B_2.CMP", "PWM.MAX"="PWM.B_2.MAX", "DIO/PWM"=refnum<k21> "ConnectorB/DIO10", "SELECT"=w383) -> ("DIO.IN"=w329:bool, "PWM.CNTR"=→"PWM.B_2.CNTR":u16)  [unwired: 10 in]
    n155 = call "DIO_Encoder.vi"("DIO.1:0.OUT"=w338, "DIO.1:0.DIR"=w333, "QE.CNFG"="ENC.B.CNFG", "DIO.1/QE.B"=refnum<k21> "ConnectorB/DIO12", "SELECT"=w382, "DIO.0/QE.A"=refnum<k21> "ConnectorB/DIO11") -> ("DIO.1:0.IN"=w328:fxp<+,2,2>, "QE.CNTR"=→"ENC.B.CNTR":u32, "QE.STAT"=→"ENC.B.STAT":u8)  [unwired: 11 in]
    n156 = call "DIO 1-bit.vi"("DIR"=w332, "OUT"=w337, "DIO Refnum"=refnum<k21> "ConnectorB/DIO13") -> ("IN"=w327:bool)  [unwired: 8 in]
    n157 = call "DIO_I2C.vi"("DIO.1:0.OUT"=w389, "DIO.1:0.DIR"=w388, "I2C.CNFG"="I2C.B.CNFG", "I2C.CNTL"="I2C.B.CNTL", "I2C.ADDR"="I2C.B.ADDR", "I2C.DATO"="I2C.B.DATO", "DIO.1/I2C.SDA"=refnum<k21> "ConnectorB/DIO15" ("DIO.1/I2C.SCL"), "I2C.CNTR"="I2C.B.CNTR", "DIO.0/I2C.SCL"=refnum<k21> "ConnectorB/DIO14" ("DIO.0/I2C.SDA"), "Execute?"="I2C.B.GO", "SELECT"=w381) -> ("DIO.1:0.IN"=w387:fxp<+,2,2>, "I2C.DATI"=→"I2C.B.DATI":u8, "I2C.STAT"=→"I2C.B.STAT":u8)  [unwired: 6 in]
    n158 = call "Join HDC Bank2 DIO.vi"("IN 7:6"=w387, "IN 5"=w327, "IN 4:3"=w328, "IN 0"=w331, "IN 2"=w329, "IN 1"=w330) -> ("OUT 7:0"=→"DIO.B_15:8.IN":u8)  [unwired: 4 in]
  }
  n159 = node-c288(w3) -> ()
  n160 = node-c288() -> (w8:T2)  [unwired: 1 in]
  n161 = timed-loop {
    timing: w8 -> [_]
    timing-out: [_] -> w7
    stop <- FALSE stop-if-true
    n162 = call "Split myDAQ DIO.vi"("IN 7:0"="DIO.C_7:0.OUT") -> ("OUT 2, OUT0"=w436:fxp<+,2,2>, "OUT 1"=w435:bool, "OUT 3"=w434:bool, "OUT 7"=w431:bool, "OUT 6, OUT 4"=w433:fxp<+,2,2>, "OUT 5"=w432:bool)  [unwired: 4 in]
    n163 = call "Split myDAQ DIO.vi"("IN 7:0"="DIO.C_7:0.DIR") -> ("OUT 2, OUT0"=w430:fxp<+,2,2>, "OUT 1"=w429:bool, "OUT 3"=w428:bool, "OUT 7"=w425:bool, "OUT 6, OUT 4"=w427:fxp<+,2,2>, "OUT 5"=w426:bool)  [unwired: 4 in]
    n164 = call "Split myDAQ Function Select.vi"("IN 7:0"="SYS.SELECTC") -> ("OUT 0"=w442:bool, "OUT 1"=w441:bool, "OUT 2"=w440:bool, "OUT 3"=w439:bool)  [unwired: 2 in]
    n165 = call "DIO_Encoder.vi"("DIO.1:0.OUT"=w436, "DIO.1:0.DIR"=w430, "QE.CNFG"="ENC.C_0.CNFG", "DIO.1/QE.B"=refnum<k21> "ConnectorC/DIO2", "SELECT"=w442, "DIO.0/QE.A"=refnum<k21> "ConnectorC/DIO0") -> ("DIO.1:0.IN"=w423:fxp<+,2,2>, "QE.CNTR"=→"ENC.C_0.CNTR":u32, "QE.STAT"=→"ENC.C_0.STAT":u8)  [unwired: 11 in]
    n166 = call "DIO 1-bit.vi"("DIR"=w429, "OUT"=w435, "DIO Refnum"=refnum<k21> "ConnectorC/DIO1") -> ("IN"=w422:bool)  [unwired: 8 in]
    n167 = call "DIO_PWM.vi"("DIO.OUT"=w434, "DIO.DIR"=w428, "PWM.CS"="PWM.C_0.CS", "PWM.CNFG"="PWM.C_0.CNFG", "PWM.CMP"="PWM.C_0.CMP", "PWM.MAX"="PWM.C_0.MAX", "DIO/PWM"=refnum<k21> "ConnectorC/DIO3", "SELECT"=w441) -> ("DIO.IN"=w421:bool, "PWM.CNTR"=→"PWM.C_0.CNTR":u16)  [unwired: 10 in]
    n168 = call "DIO_Encoder.vi"("DIO.1:0.OUT"=w433, "DIO.1:0.DIR"=w427, "QE.CNFG"="ENC.C_1.CNFG", "DIO.1/QE.B"=refnum<k21> "ConnectorC/DIO6", "SELECT"=w440, "DIO.0/QE.A"=refnum<k21> "ConnectorC/DIO4") -> ("DIO.1:0.IN"=w420:fxp<+,2,2>, "QE.CNTR"=→"ENC.C_1.CNTR":u32, "QE.STAT"=→"ENC.C_1.STAT":u8)  [unwired: 11 in]
    n169 = call "DIO 1-bit.vi"("DIR"=w426, "OUT"=w432, "DIO Refnum"=refnum<k21> "ConnectorC/DIO5") -> ("IN"=w419:bool)  [unwired: 8 in]
    n170 = call "DIO_PWM.vi"("DIO.OUT"=w431, "DIO.DIR"=w425, "PWM.CS"="PWM.C_1.CS", "PWM.CNFG"="PWM.C_1.CNFG", "PWM.CMP"="PWM.C_1.CMP", "PWM.MAX"="PWM.C_1.MAX", "DIO/PWM"=refnum<k21> "ConnectorC/DIO7", "SELECT"=w439) -> ("DIO.IN"=w418:bool, "PWM.CNTR"=→"PWM.C_1.CNTR":u16)  [unwired: 10 in]
    n171 = call "Join myDAQ DIO.vi"("IN 7"=w418, "IN 5"=w419, "IN 6, IN 4"=w420, "IN 2, IN 0"=w423, "IN 3"=w421, "IN 1"=w422) -> ("IN 7:0"=→"DIO.C_7:0.IN":u8)  [unwired: 4 in]
  }
  n172 = node-c288(w7) -> ()
